vi "PYBD<-> Keyboard.vi"() -> ()   [LabVIEW 2019]
uses:
  <userlib>/MicroPython/VIs/uPythonX/uPythonX.xctl
panel:
  in  "KeyLUT":T1(xcontrol)={"Port"="PyBoard - ASRL44::INSTR", "All Code"="PLAIN = 0x00\nSHIFT = 0x02\nkbmap = dict()\nkbmap['LCTRL'] = (0x01,PLAIN)\nkbmap['LSHIFT'] = (0x02,PLAIN)\nkbmap['LALT'] = (0x04,PLAIN)\nkbmap['LMETA'] = (0x08,PLAIN)\nkbmap['RCTRL'] = (0x10,PLAIN)\nkbmap['RSHIFT'] = (0x20,PLAIN)\nkbmap['RALT'] = (0x40,PLAIN)\nkbmap['RMETA'] = (0x80,PLAIN)\nkbmap['NONE'] = (0x00,PLAIN)\nkbmap['ERR_OVF'] = (0x01,PLAIN)\nkbmap['a'] = (0x04,PLAIN)\nkbmap['A'] = (0x04,SHIFT)\nkbmap['b'] = (0x05,PLAIN)\nkbmap['B'] = (0x05,SHIFT)\nkbmap['c'] = (0x06,PLAIN)\nkbmap['C'] = (0x06,SHIFT)\nkbmap['d'] = (0x07,PLAIN)\nkbmap['D'] = (0x07,SHIFT)\nkbmap['e'] = (0x08,PLAIN)\nkbmap['E'] = (0x08,SHIFT)\nkbmap['f'] = (0x09,PLAIN)\nkbmap['F'] = (0x09,SHIFT)\nkbmap['g'] = (0x0a,PLAIN)\nkbmap['G'] = (0x0a,SHIFT)\nkbmap['h'] = (0x0b,PLAIN)\nkbmap['H'] = (0x0b,SHIFT)\nkbmap['i'] = (0x0c,PLAIN)\nkbmap['I'] = (0x0c,SHIFT)\nkbmap['j'] = (0x0d,PLAIN)\nkbmap['J'] = (0x0d,SHIFT)\nkbmap['k'] = (0x0e,PLAIN)\nkbmap['K'] = (0x0e,SHIFT)\nkbmap['l'] = (0x0f,PLAIN)\nkbmap['L'] = (0x0f,SHIFT)\nkbmap['m'] = (0x10,PLAIN)\nkbmap['M'] = (0x10,SHIFT)\nkbmap['n'] = (0x11,PLAIN)\nkbmap['N'] = (0x11,SHIFT)\nkbmap['o'] = (0x12,PLAIN)\nkbmap['O'] = (0x12,SHIFT)\nkbmap['p'] = (0x13,PLAIN)\nkbmap['P'] = (0x13,SHIFT)\nkbmap['q'] = (0x14,PLAIN)\nkbmap['Q'] = (0x14,SHIFT)\nkbmap['r'] = (0x15,PLAIN)\nkbmap['R'] = (0x15,SHIFT)\nkbmap['s'] = (0x16,PLAIN)\nkbmap['S'] = (0x16,SHIFT)\nkbmap['t'] = (0x17,PLAIN)\nkbmap['T'] = (0x17,SHIFT)\nkbmap['u'] = (0x18,PLAIN)\nkbmap['U'] = (0x18,SHIFT)\nkbmap['v'] = (0x19,PLAIN)\nkbmap['V'] = (0x19,SHIFT)\nkbmap['w'] = (0x1a,PLAIN)\nkbmap['W'] = (0x1a,SHIFT)\nkbmap['x'] = (0x1b,PLAIN)\nkbmap['X'] = (0x1b,SHIFT)\nkbmap['y'] = (0x1c,PLAIN)\nkbmap['Y'] = (0x1c,SHIFT)\nkbmap['z'] = (0x1d,PLAIN)\nkbmap['Z'] = (0x1d,SHIFT)\nkbmap['1'] = (0x1e,PLAIN)\nkbmap['!'] = (0x1e,SHIFT)\nkbmap['2'] = (0x1f,PLAIN)\nkbmap['@'] = (0x1f,SHIFT)\nkbmap['3'] = (0x20,PLAIN)\nkbmap['#'] = (0x20,SHIFT)\nkbmap['4'] = (0x21,PLAIN)\nkbmap['$'] = (0x21,SHIFT)\nkbmap['5'] = (0x22,PLAIN)\nkbmap['%'] = (0x22,SHIFT)\nkbmap['6'] = (0x23,PLAIN)\nkbmap['^'] = (0x23,SHIFT)\nkbmap['7'] = (0x24,PLAIN)\nkbmap['&'] = (0x24,SHIFT)\nkbmap['8'] = (0x25,PLAIN)\nkbmap['*'] = (0x25,SHIFT)\nkbmap['9'] = (0x26,PLAIN)\nkbmap['('] = (0x26,SHIFT)\nkbmap['0'] = (0x27,PLAIN)\nkbmap[')'] = (0x27,SHIFT)\nkbmap['ENTER'] = (0x28,PLAIN)\nkbmap['ESC'] = (0x29,PLAIN)\nkbmap['BACKSPACE'] = (0x2a,PLAIN)\nkbmap['\\t'] = (0x2b,PLAIN)\nkbmap[' '] = (0x2c,PLAIN)\nkbmap['-'] = (0x2d,PLAIN)\nkbmap['_'] = (0x2d,SHIFT)\nkbmap['='] = (0x2e,PLAIN)\nkbmap['+'] = (0x2e,SHIFT)\nkbmap['['] = (0x2f,PLAIN)\nkbmap['{'] = (0x2f,SHIFT)\nkbmap[']'] = (0x30,PLAIN)\nkbmap['}'] = (0x30,SHIFT)\nkbmap['\\\\'] = (0x31,PLAIN)\nkbmap['|'] = (0x31,SHIFT)\nkbmap['~'] = (0x32,PLAIN)\nkbmap[';'] = (0x33,PLAIN)\nkbmap[':'] = (0x33,SHIFT)\nkbmap[\"'\"] = (0x34,PLAIN)\nkbmap['\"'] = (0x34,SHIFT)\nkbmap['GRAVE'] = (0x35,PLAIN)\nkbmap[','] = (0x36,PLAIN)\nkbmap['<'] = (0x36,SHIFT)\nkbmap['.'] = (0x37,PLAIN)\nkbmap['>'] = (0x37,SHIFT)\nkbmap['/'] = (0x38,PLAIN)\nkbmap['?'] = (0x38,SHIFT)\nkbmap['CAPSLOCK'] = (0x39,PLAIN)\nkbmap['F1'] = (0x3a,PLAIN)\nkbmap['F2'] = (0x3b,PLAIN)\nkbmap['F3'] = (0x3c,PLAIN)\nkbmap['F4'] = (0x3d,PLAIN)\nkbmap['F5'] = (0x3e,PLAIN)\nkbmap['F6'] = (0x3f,PLAIN)\nkbmap['F7'] = (0x40,PLAIN)\nkbmap['F8'] = (0x41,PLAIN)\nkbmap['F9'] = (0x42,PLAIN)\nkbmap['F10'] = (0x43,PLAIN)\nkbmap['F11'] = (0x44,PLAIN)\nkbmap['F12'] = (0x45,PLAIN)\nkbmap['SYSRQ'] = (0x46,PLAIN)\nkbmap['SCROLLLOCK'] = (0x47,PLAIN)\nkbmap['PAUSE'] = (0x48,PLAIN)\nkbmap['INSERT'] = (0x49,PLAIN)\nkbmap['HOME'] = (0x4a,PLAIN)\nkbmap['PAGEUP'] = (0x4b,PLAIN)\nkbmap['DELETE'] = (0x4c,PLAIN)\nkbmap['END'] = (0x4d,PLAIN)\nkbmap['PAGEDOWN'] = (0x4e,PLAIN)\nkbmap['RIGHT'] = (0x4f,PLAIN)\nkbmap['LEFT'] = (0x50,PLAIN)\nkbmap['DOWN'] = (0x51,PLAIN)\nkbmap['UP'] = (0x52,PLAIN)\nkbmap['NUMLOCK'] = (0x53,PLAIN)\nkbmap['F13'] = (0x68,PLAIN)\nkbmap['F14'] = (0x69,PLAIN)\nkbmap['F15'] = (0x6a,PLAIN)\nkbmap['F16'] = (0x6b,PLAIN)\nkbmap['F17'] = (0x6c,PLAIN)\nkbmap['F18'] = (0x6d,PLAIN)\nkbmap['F19'] = (0x6e,PLAIN)\nkbmap['F20'] = (0x6f,PLAIN)\nkbmap['F21'] = (0x70,PLAIN)\nkbmap['F22'] = (0x71,PLAIN)\nkbmap['F23'] = (0x72,PLAIN)\nkbmap['F24'] = (0x73,PLAIN)\nkbmap['OPEN'] = (0x74,PLAIN)\nkbmap['HELP'] = (0x75,PLAIN)\nkbmap['PROPS'] = (0x76,PLAIN)\nkbmap['FRONT'] = (0x77,PLAIN)\nkbmap['STOP'] = (0x78,PLAIN)\nkbmap['AGAIN'] = (0x79,PLAIN)\nkbmap['UNDO'] = (0x7a,PLAIN)\nkbmap['CUT'] = (0x7b,PLAIN)\nkbmap['COPY'] = (0x7c,PLAIN)\nkbmap['PASTE'] = (0x7d,PLAIN)\nkbmap['FIND'] = (0x7e,PLAIN)\nkbmap['MUTE'] = (0x7f,PLAIN)\nkbmap['VOLUMEUP'] = (0x80,PLAIN)\nkbmap['VOLUMEDOWN'] = (0x81,PLAIN)"}
  out "regular expression":string="PLAIN = 0x00\nSHIFT = 0x02\nkbmap = dict()\nkbmap['MOD_LCTRL'] = (0x01,PLAIN)\nkbmap['MOD_LSHIFT'] = (0x02,PLAIN)\nkbmap['MOD_LALT'] = (0x04,PLAIN)\nkbmap['MOD_LMETA'] = (0x08,PLAIN)\nkbmap['MOD_RCTRL'] = (0x10,PLAIN)\nkbmap['MOD_RSHIFT'] = (0x20,PLAIN)\nkbmap['MOD_RALT'] = (0x40,PLAIN)\nkbmap['MOD_RMETA'] = (0x80,PLAIN)\nkbmap['NONE'] = (0x00,PLAIN)\nkbmap['ERR_OVF'] = (0x01,PLAIN)\nkbmap['a'] = (0x04,PLAIN)\nkbmap['A'] = (0x04,SHIFT)\nkbmap['b'] = (0x05,PLAIN)\nkbmap['B'] = (0x05,SHIFT)\nkbmap['c'] = (0x06,PLAIN)\nkbmap['C'] = (0x06,SHIFT)\nkbmap['d'] = (0x07,PLAIN)\nkbmap['D'] = (0x07,SHIFT)\nkbmap['e'] = (0x08,PLAIN)\nkbmap['E'] = (0x08,SHIFT)\nkbmap['f'] = (0x09,PLAIN)\nkbmap['F'] = (0x09,SHIFT)\nkbmap['g'] = (0x0a,PLAIN)\nkbmap['G'] = (0x0a,SHIFT)\nkbmap['h'] = (0x0b,PLAIN)\nkbmap['H'] = (0x0b,SHIFT)\nkbmap['i'] = (0x0c,PLAIN)\nkbmap['I'] = (0x0c,SHIFT)\nkbmap['j'] = (0x0d,PLAIN)\nkbmap['J'] = (0x0d,SHIFT)\nkbmap['k'] = (0x0e,PLAIN)\nkbmap['K'] = (0x0e,SHIFT)\nkbmap['l'] = (0x0f,PLAIN)\nkbmap['L'] = (0x0f,SHIFT)\nkbmap['m'] = (0x10,PLAIN)\nkbmap['M'] = (0x10,SHIFT)\nkbmap['n'] = (0x11,PLAIN)\nkbmap['N'] = (0x11,SHIFT)\nkbmap['o'] = (0x12,PLAIN)\nkbmap['O'] = (0x12,SHIFT)\nkbmap['p'] = (0x13,PLAIN)\nkbmap['P'] = (0x13,SHIFT)\nkbmap['q'] = (0x14,PLAIN)\nkbmap['Q'] = (0x14,SHIFT)\nkbmap['r'] = (0x15,PLAIN)\nkbmap['R'] = (0x15,SHIFT)\nkbmap['s'] = (0x16,PLAIN)\nkbmap['S'] = (0x16,SHIFT)\nkbmap['t'] = (0x17,PLAIN)\nkbmap['T'] = (0x17,SHIFT)\nkbmap['u'] = (0x18,PLAIN)\nkbmap['U'] = (0x18,SHIFT)\nkbmap['v'] = (0x19,PLAIN)\nkbmap['V'] = (0x19,SHIFT)\nkbmap['w'] = (0x1a,PLAIN)\nkbmap['W'] = (0x1a,SHIFT)\nkbmap['x'] = (0x1b,PLAIN)\nkbmap['X'] = (0x1b,SHIFT)\nkbmap['y'] = (0x1c,PLAIN)\nkbmap['Y'] = (0x1c,SHIFT)\nkbmap['z'] = (0x1d,PLAIN)\nkbmap['Z'] = (0x1d,SHIFT)\nkbmap['1'] = (0x1e,PLAIN)\nkbmap['1'] = (0x1e,SHIFT)\nkbmap['2'] = (0x1f,PLAIN)\nkbmap['2'] = (0x1f,SHIFT)\nkbmap['3'] = (0x20,PLAIN)\nkbmap['3'] = (0x20,SHIFT)\nkbmap['4'] = (0x21,PLAIN)\nkbmap['4'] = (0x21,SHIFT)\nkbmap['5'] = (0x22,PLAIN)\nkbmap['5'] = (0x22,SHIFT)\nkbmap['6'] = (0x23,PLAIN)\nkbmap['6'] = (0x23,SHIFT)\nkbmap['7'] = (0x24,PLAIN)\nkbmap['7'] = (0x24,SHIFT)\nkbmap['8'] = (0x25,PLAIN)\nkbmap['8'] = (0x25,SHIFT)\nkbmap['9'] = (0x26,PLAIN)\nkbmap['9'] = (0x26,SHIFT)\nkbmap['0'] = (0x27,PLAIN)\nkbmap['0'] = (0x27,SHIFT)\nkbmap['ENTER'] = (0x28,PLAIN)\nkbmap['ESC'] = (0x29,PLAIN)\nkbmap['BACKSPACE'] = (0x2a,PLAIN)\nkbmap['TAB'] = (0x2b,PLAIN)\nkbmap['SPACE'] = (0x2c,PLAIN)\nkbmap['MINUS'] = (0x2d,PLAIN)\nkbmap['EQUAL'] = (0x2e,PLAIN)\nkbmap['LEFTBRACE'] = (0x2f,PLAIN)\nkbmap['RIGHTBRACE'] = (0x30,PLAIN)\nkbmap['BACKSLASH'] = (0x31,PLAIN)\nkbmap['HASHTILDE'] = (0x32,PLAIN)\nkbmap['SEMICOLON'] = (0x33,PLAIN)\nkbmap['APOSTROPHE'] = (0x34,PLAIN)\nkbmap['GRAVE'] = (0x35,PLAIN)\nkbmap['COMMA'] = (0x36,PLAIN)\nkbmap['DOT'] = (0x37,PLAIN)\nkbmap['SLASH'] = (0x38,PLAIN)\nkbmap['CAPSLOCK'] = (0x39,PLAIN)\nkbmap['F'] = (0x3a,PLAIN)\nkbmap['1'] = (0x3a,SHIFT)\nkbmap['F'] = (0x3b,PLAIN)\nkbmap['2'] = (0x3b,SHIFT)\nkbmap['F'] = (0x3c,PLAIN)\nkbmap['3'] = (0x3c,SHIFT)\nkbmap['F'] = (0x3d,PLAIN)\nkbmap['4'] = (0x3d,SHIFT)\nkbmap['F'] = (0x3e,PLAIN)\nkbmap['5'] = (0x3e,SHIFT)\nkbmap['F'] = (0x3f,PLAIN)\nkbmap['6'] = (0x3f,SHIFT)\nkbmap['F'] = (0x40,PLAIN)\nkbmap['7'] = (0x40,SHIFT)\nkbmap['F'] = (0x41,PLAIN)\nkbmap['8'] = (0x41,SHIFT)\nkbmap['F'] = (0x42,PLAIN)\nkbmap['9'] = (0x42,SHIFT)\nkbmap['F10'] = (0x43,PLAIN)\nkbmap['F11'] = (0x44,PLAIN)\nkbmap['F12'] = (0x45,PLAIN)\nkbmap['SYSRQ'] = (0x46,PLAIN)\nkbmap['SCROLLLOCK'] = (0x47,PLAIN)\nkbmap['PAUSE'] = (0x48,PLAIN)\nkbmap['INSERT'] = (0x49,PLAIN)\nkbmap['HOME'] = (0x4a,PLAIN)\nkbmap['PAGEUP'] = (0x4b,PLAIN)\nkbmap['DELETE'] = (0x4c,PLAIN)\nkbmap['END'] = (0x4d,PLAIN)\nkbmap['PAGEDOWN'] = (0x4e,PLAIN)\nkbmap['RIGHT'] = (0x4f,PLAIN)\nkbmap['LEFT'] = (0x50,PLAIN)\nkbmap['DOWN'] = (0x51,PLAIN)\nkbmap['U'] = (0x52,PLAIN)\nkbmap['P'] = (0x52,SHIFT)\nkbmap['NUMLOCK'] = (0x53,PLAIN)\nkbmap['KPSLASH'] = (0x54,PLAIN)\nkbmap['KPASTERISK'] = (0x55,PLAIN)\nkbmap['KPMINUS'] = (0x56,PLAIN)\nkbmap['KPPLUS'] = (0x57,PLAIN)\nkbmap['KPENTER'] = (0x58,PLAIN)\nkbmap['KP1'] = (0x59,PLAIN)\nkbmap['KP2'] = (0x5a,PLAIN)\nkbmap['KP3'] = (0x5b,PLAIN)\nkbmap['KP4'] = (0x5c,PLAIN)\nkbmap['KP5'] = (0x5d,PLAIN)\nkbmap['KP6'] = (0x5e,PLAIN)\nkbmap['KP7'] = (0x5f,PLAIN)\nkbmap['KP8'] = (0x60,PLAIN)\nkbmap['KP9'] = (0x61,PLAIN)\nkbmap['KP0'] = (0x62,PLAIN)\nkbmap['KPDOT'] = (0x63,PLAIN)\nkbmap['102ND'] = (0x64,PLAIN)\nkbmap['COMPOSE'] = (0x65,PLAIN)\nkbmap['POWER'] = (0x66,PLAIN)\nkbmap['KPEQUAL'] = (0x67,PLAIN)\nkbmap['F13'] = (0x68,PLAIN)\nkbmap['F14'] = (0x69,PLAIN)\nkbmap['F15'] = (0x6a,PLAIN)\nkbmap['F16'] = (0x6b,PLAIN)\nkbmap['F17'] = (0x6c,PLAIN)\nkbmap['F18'] = (0x6d,PLAIN)\nkbmap['F19'] = (0x6e,PLAIN)\nkbmap['F20'] = (0x6f,PLAIN)\nkbmap['F21'] = (0x70,PLAIN)\nkbmap['F22'] = (0x71,PLAIN)\nkbmap['F23'] = (0x72,PLAIN)\nkbmap['F24'] = (0x73,PLAIN)\nkbmap['OPEN'] = (0x74,PLAIN)\nkbmap['HELP'] = (0x75,PLAIN)\nkbmap['PROPS'] = (0x76,PLAIN)\nkbmap['FRONT'] = (0x77,PLAIN)\nkbmap['STOP'] = (0x78,PLAIN)\nkbmap['AGAIN'] = (0x79,PLAIN)\nkbmap['UNDO'] = (0x7a,PLAIN)\nkbmap['CUT'] = (0x7b,PLAIN)\nkbmap['COPY'] = (0x7c,PLAIN)\nkbmap['PASTE'] = (0x7d,PLAIN)\nkbmap['FIND'] = (0x7e,PLAIN)\nkbmap['MUTE'] = (0x7f,PLAIN)\nkbmap['VOLUMEUP'] = (0x80,PLAIN)\nkbmap['VOLUMEDOWN'] = (0x81,PLAIN)\n"
  out "Table Control":string[][](table)=[["MOD_LCTRL", "0x01", ""], ["MOD_LSHIFT", "0x02", ""], ["MOD_LALT", "0x04", ""], ["MOD_LMETA", "0x08", ""], ["MOD_RCTRL", "0x10", ""], ["MOD_RSHIFT", "0x20", ""], ["MOD_RALT", "0x40", ""], ["MOD_RMETA", "0x80", ""], ["NONE", "0x00", "No key pressed"], ["ERR_OVF", "0x01", "Keyboard Error Roll Over - used for all slots if too many keys are pressed (\"Phantom key\")"], ["A", "0x04", "Keyboard a and A"], ["B", "0x05", "Keyboard b and B"], ["C", "0x06", "Keyboard c and C"], ["D", "0x07", "Keyboard d and D"], ["E", "0x08", "Keyboard e and E"], ["F", "0x09", "Keyboard f and F"], ["G", "0x0a", "Keyboard g and G"], ["H", "0x0b", "Keyboard h and H"], ["I", "0x0c", "Keyboard i and I"], ["J", "0x0d", "Keyboard j and J"], ["K", "0x0e", "Keyboard k and K"], ["L", "0x0f", "Keyboard l and L"], ["M", "0x10", "Keyboard m and M"], ["N", "0x11", "Keyboard n and N"], ["O", "0x12", "Keyboard o and O"], ["P", "0x13", "Keyboard p and P"], ["Q", "0x14", "Keyboard q and Q"], ["R", "0x15", "Keyboard r and R"], ["S", "0x16", "Keyboard s and S"], ["T", "0x17", "Keyboard t and T"], ["U", "0x18", "Keyboard u and U"], ["V", "0x19", "Keyboard v and V"], ["W", "0x1a", "Keyboard w and W"], ["X", "0x1b", "Keyboard x and X"], ["Y", "0x1c", "Keyboard y and Y"], ["Z", "0x1d", "Keyboard z and Z"], ["1", "0x1e", "Keyboard 1 and !"], ["2", "0x1f", "Keyboard 2 and @"], ["3", "0x20", "Keyboard 3 and #"], ["4", "0x21", "Keyboard 4 and $"], ["5", "0x22", "Keyboard 5 and %"], ["6", "0x23", "Keyboard 6 and ^"], ["7", "0x24", "Keyboard 7 and &"], ["8", "0x25", "Keyboard 8 and *"], ["9", "0x26", "Keyboard 9 and ("], ["0", "0x27", "Keyboard 0 and )"], ["ENTER", "0x28", "Keyboard Return (ENTER)"], ["ESC", "0x29", "Keyboard ESCAPE"], ["BACKSPACE", "0x2a", "Keyboard DELETE (Backspace)"], ["TAB", "0x2b", "Keyboard Tab"], ["SPACE", "0x2c", "Keyboard Spacebar"], ["MINUS", "0x2d", "Keyboard - and _"], ["EQUAL", "0x2e", "Keyboard = and +"], ["LEFTBRACE", "0x2f", "Keyboard [ and {"], ["RIGHTBRACE", "0x30", "Keyboard ] and }"], ["BACKSLASH", "0x31", "Keyboard \\ and |"], ["HASHTILDE", "0x32", "Keyboard Non-US # and ~"], ["SEMICOLON", "0x33", "Keyboard ; and :"], ["APOSTROPHE", "0x34", "Keyboard ' and \""], ["GRAVE", "0x35", "Keyboard ` and ~"], ["COMMA", "0x36", "Keyboard , and <"], ["DOT", "0x37", "Keyboard . and >"], ["SLASH", "0x38", "Keyboard / and ?"], ["CAPSLOCK", "0x39", "Keyboard Caps Lock"], ["F1", "0x3a", "Keyboard F1"], ["F2", "0x3b", "Keyboard F2"], ["F3", "0x3c", "Keyboard F3"], ["F4", "0x3d", "Keyboard F4"], ["F5", "0x3e", "Keyboard F5"], ["F6", "0x3f", "Keyboard F6"], ["F7", "0x40", "Keyboard F7"], ["F8", "0x41", "Keyboard F8"], ["F9", "0x42", "Keyboard F9"], ["F10", "0x43", "Keyboard F10"], ["F11", "0x44", "Keyboard F11"], ["F12", "0x45", "Keyboard F12"], ["SYSRQ", "0x46", "Keyboard Print Screen"], ["SCROLLLOCK", "0x47", "Keyboard Scroll Lock"], ["PAUSE", "0x48", "Keyboard Pause"], ["INSERT", "0x49", "Keyboard Insert"], ["HOME", "0x4a", "Keyboard Home"], ["PAGEUP", "0x4b", "Keyboard Page Up"], ["DELETE", "0x4c", "Keyboard Delete Forward"], ["END", "0x4d", "Keyboard End"], ["PAGEDOWN", "0x4e", "Keyboard Page Down"], ["RIGHT", "0x4f", "Keyboard Right Arrow"], ["LEFT", "0x50", "Keyboard Left Arrow"], ["DOWN", "0x51", "Keyboard Down Arrow"], ["UP", "0x52", "Keyboard Up Arrow"], ["NUMLOCK", "0x53", "Keyboard Num Lock and Clear"], ["KPSLASH", "0x54", "Keypad /"], ["KPASTERISK", "0x55", "Keypad *"], ["KPMINUS", "0x56", "Keypad -"], ["KPPLUS", "0x57", "Keypad +"], ["KPENTER", "0x58", "Keypad ENTER"], ["KP1", "0x59", "Keypad 1 and End"], ["KP2", "0x5a", "Keypad 2 and Down Arrow"], ["KP3", "0x5b", "Keypad 3 and PageDn"], ["KP4", "0x5c", "Keypad 4 and Left Arrow"], ["KP5", "0x5d", "Keypad 5"], ["KP6", "0x5e", "Keypad 6 and Right Arrow"], ["KP7", "0x5f", "Keypad 7 and Home"], ["KP8", "0x60", "Keypad 8 and Up Arrow"], ["KP9", "0x61", "Keypad 9 and Page Up"], ["KP0", "0x62", "Keypad 0 and Insert"], ["KPDOT", "0x63", "Keypad . and Delete"], ["102ND", "0x64", "Keyboard Non-US \\ and |"], ["COMPOSE", "0x65", "Keyboard Application"], ["POWER", "0x66", "Keyboard Power"], ["KPEQUAL", "0x67", "Keypad ="], ["F13", "0x68", "Keyboard F13"], ["F14", "0x69", "Keyboard F14"], ["F15", "0x6a", "Keyboard F15"], ["F16", "0x6b", "Keyboard F16"], ["F17", "0x6c", "Keyboard F17"], ["F18", "0x6d", "Keyboard F18"], ["F19", "0x6e", "Keyboard F19"], ["F20", "0x6f", "Keyboard F20"], ["F21", "0x70", "Keyboard F21"], ["F22", "0x71", "Keyboard F22"], ["F23", "0x72", "Keyboard F23"], ["F24", "0x73", "Keyboard F24"], ["OPEN", "0x74", "Keyboard Execute"], ["HELP", "0x75", "Keyboard Help"], ["PROPS", "0x76", "Keyboard Menu"], ["FRONT", "0x77", "Keyboard Select"], ["STOP", "0x78", "Keyboard Stop"], ["AGAIN", "0x79", "Keyboard Again"], ["UNDO", "0x7a", "Keyboard Undo"], ["CUT", "0x7b", "Keyboard Cut"], ["COPY", "0x7c", "Keyboard Copy"], ["PASTE", "0x7d", "Keyboard Paste"], ["FIND", "0x7e", "Keyboard Find"], ["MUTE", "0x7f", "Keyboard Mute"], ["VOLUMEUP", "0x80", "Keyboard Volume Up"], ["VOLUMEDOWN", "0x81", "Keyboard Volume Downe"]]
  in  "uPythonX":T1(xcontrol)={"Port"="PyBoard - ASRL44::INSTR", "All Code"="'''\nhttp://wiki.micropython.org/USB-HID-Keyboard-mode-example-a-password-dongle\n     \n#boot.py\nimport machine\nimport pyb\n#pyb.main('main.py') # main script to run after this one\n#pyb.usb_mode('CDC+MSC') # act as a serial and a storage device\npyb.usb_mode('CDC+HID',hid=pyb.hid_keyboard)\n\nFor arduino - https://www.sparkfun.com/tutorials/337\n'''\n\nimport pyb,utime\nimport KeyLUT\nkb = pyb.USB_HID()\nbuf = bytearray(8)\n# Sending T\n# Do the key down\ndef typeKey(letter):\n     \n     buf[0] = KeyLUT.kbmap[letter][1]\n     buf[2] = KeyLUT.kbmap[letter][0]\n     kb.send(buf)\n     pyb.delay(20)\n     # Do the key up\n     buf[0] = 0x00\n     buf[2] = 0x00\n     kb.send(buf)\n     pyb.delay(20)     \n\ndef typeKeys(string):\n     for letter in string:\n          typeKey(letter)\n          \ntypeKeys('!@#$%^&*(): I have a _+=-34?/<>,')"}
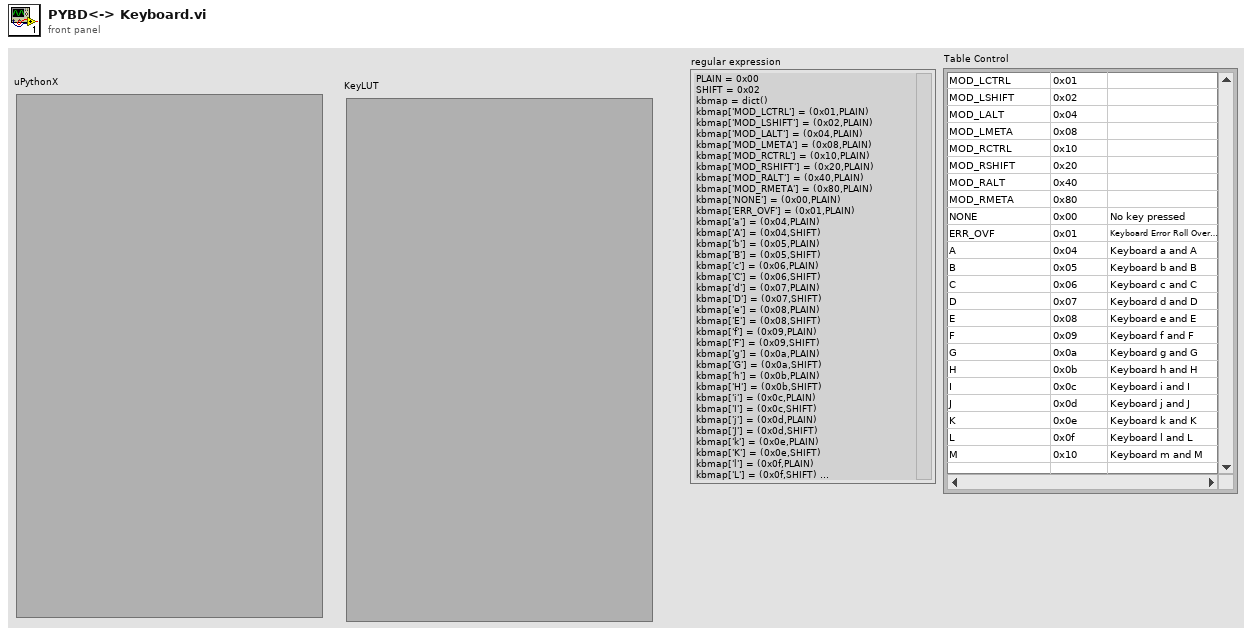
[diagram p1: front panel]
types:
  T1 = cluster{"Port":refnum<visa-resource-name>, "All Code":string}
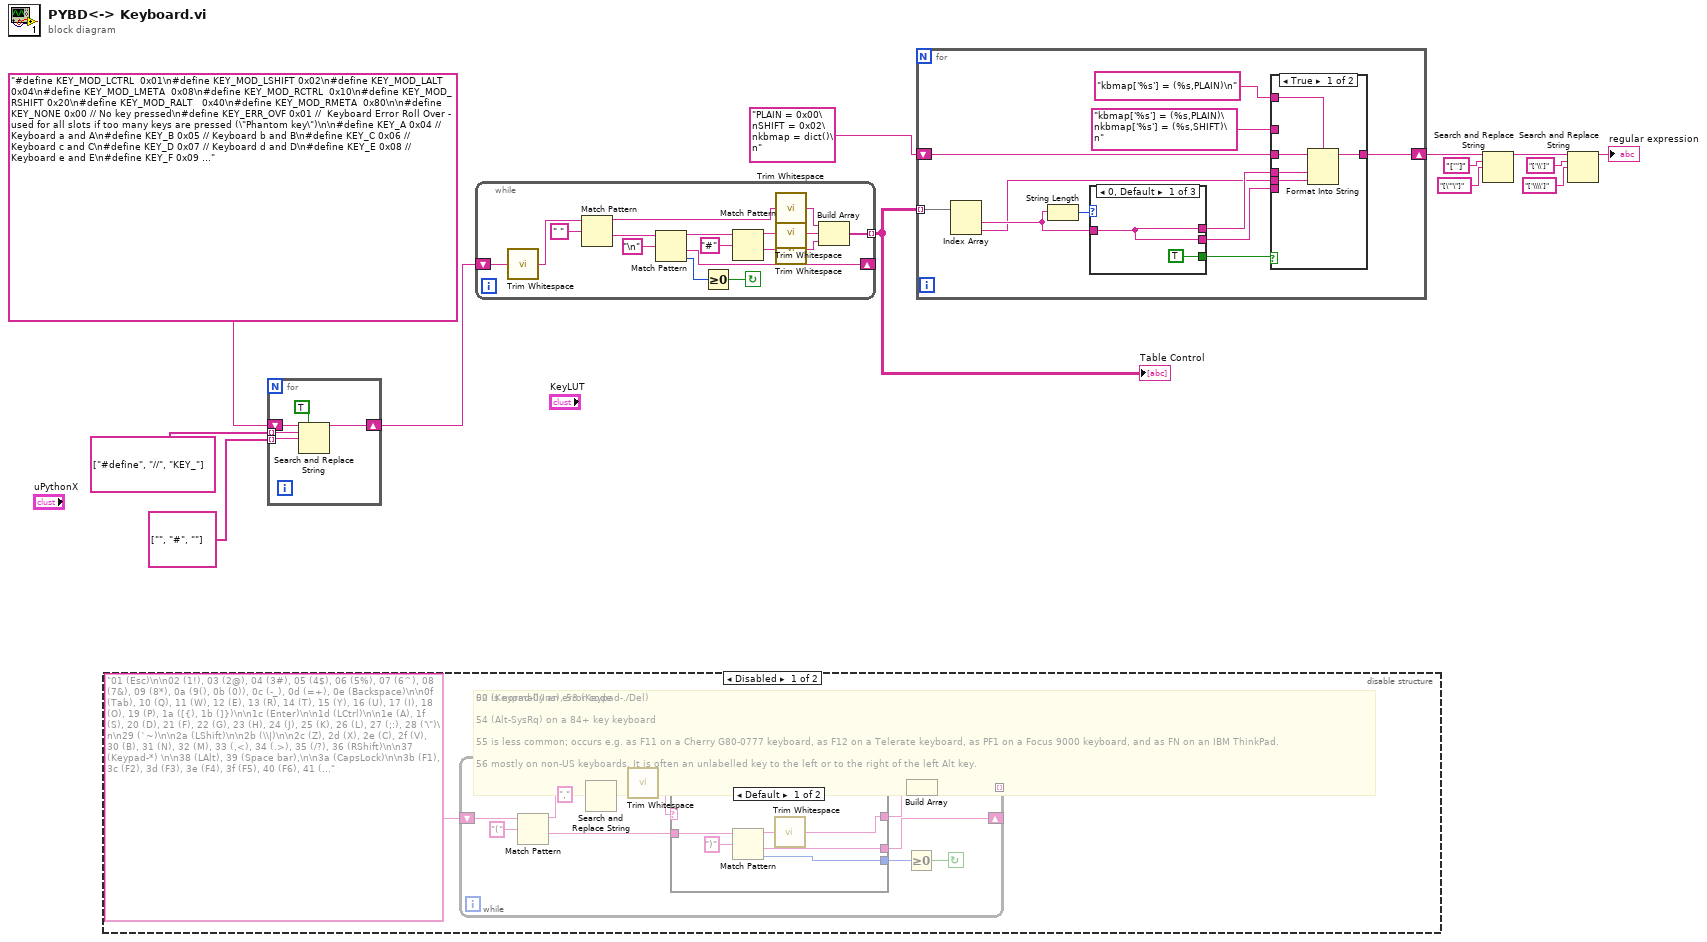
[diagram p0: block diagram]
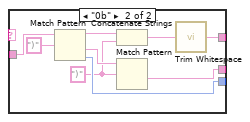
[diagram p2: hidden frame]
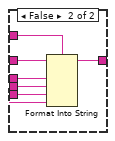
[diagram p4: hidden frame]
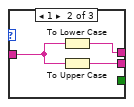
[diagram p5: hidden frame]
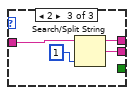
[diagram p6: hidden frame]
diagram:
  n1 = disable-structure shown="Disabled" {
    frame Disabled {
      # "00 is normally an error code"
      # "52 (Keypad-0/Ins), 53 (Keypad-./Del)\n\n54 (Alt-SysRq) on a 84+ key keyboard\n\n55 is less common; occurs e.g. as F11 on a Cherry G80-0777 keyboard, as F12 on a Telerate keyboard, as PF1 on a Focus 9000 keyboard, and as FN on an IBM ThinkPad.\n\n56 mostly on non-US keyboards. It is often an unlabelled key to the left or to the right of the left Alt key."
      n2 = while {
        shift-right: [w23] -> _
        shift-left: "01 (Esc)\n\n02 (1!), 03 (2@), 04 (3#), 05 (4$), 06 (5%), 07 (6^), 08 (7&), 09 (8*), 0a (9(), 0b (0)), 0c (-_), 0d (=+), 0e (Backspace)\n\n0f (Tab), 10 (Q), 11 (W), 12 (E), 13 (R), 14 (T), 15 (Y), 16 (U), 17 (I), 18 (O), 19 (P), 1a ([{), 1b (]})\n\n1c (Enter)\n\n1d (LCtrl)\n\n1e (A), 1f (S), 20 (D), 21 (F), 22 (G), 23 (H), 24 (J), 25 (K), 26 (L), 27 (;:), 28 ('\")\n\n29 (`~)\n\n2a (LShift)\n\n2b (\\|)\n\n2c (Z), 2d (X), 2e (C), 2f (V), 30 (B), 31 (N), 32 (M), 33 (,<), 34 (.>), 35 (/?), 36 (RShift)\n\n37 (Keypad-*) \n\n38 (LAlt), 39 (Space bar),\n\n3a (CapsLock)\n\n3b (F1), 3c (F2), 3d (F3), 3e (F4), 3f (F5), 40 (F6), 41 (F7), 42 (F8), 43 (F9), 44 (F10)\n\n45 (NumLock)\n\n46 (ScrollLock)\n\n47 (Keypad-7/Home), 48 (Keypad-8/Up), 49 (Keypad-9/PgUp)\n\n4a (Keypad--)\n\n4b (Keypad-4/Left), 4c (Keypad-5), 4d (Keypad-6/Right), 4e (Keypad-+)\n\n4f (Keypad-1/End), 50 (Keypad-2/Down), 51 (Keypad-3/PgDn)\n" ("String") -> [w26]
        tunnel: [w19] -> _ mode=indexing
        stop <- w21 continue-if-true
        n3 = Match Pattern(string=w26, regular expression="(") -> (before substring=w18:string, after substring=w24:string)  [unwired: 1 in, 2 out]
        n4 = Search and Replace String(input string=w18, search string="," ("regular expression")) -> (result string=w16:string)  [unwired: 6 in, 3 out]
        n5 = call <vilib>:"Trim Whitespace.vi"("string"=w16) -> ("trimmed string"=w15:string)  [unwired: 1 in]
        n6 = case shown="Default" w15 {
          tunnel: w24 -> [w32 w41]
          tunnel: [w29 w36] -> w23
          tunnel: [w28 w39] -> w22
          tunnel: [w27 w38] -> w20
          frame Default {
            n7 = Match Pattern(string=w32, regular expression=")") -> (before substring=w30:string, after substring=w29:string, offset past match=w28:i32)  [unwired: 1 in, 1 out]
            n8 = call <vilib>:"Trim Whitespace.vi"("string"=w30) -> ("trimmed string"=w27:string)  [unwired: 1 in]
          }
          frame "0b" {
            w34 = ")" ("regular expression")
            n9 = Match Pattern(string=w41, regular expression=")") -> (before substring=w35:string, after substring=w37:string, offset past match=w39:i32)  [unwired: 1 in, 1 out]
            n10 = Concatenate Strings(w35, w34) -> (w33:string)
            n11 = Match Pattern(string=w37, regular expression=w34) -> (after substring=w36:string)  [unwired: 1 in, 3 out]
            n12 = call <vilib>:"Trim Whitespace.vi"("string"=w33) -> ("trimmed string"=w38:string)  [unwired: 1 in]
          }
        }
        n13 = Greater Or Equal To 0?(x=w22) -> (x >= 0?=w21:bool)
        n14 = Build Array(w15, w20) -> (w19:string[])
      }
    }
    frame Enabled {
    }
  }
  n15 = for {
    tunnel: string[] ["#define", "//", "KEY_"] -> [w45] mode=indexing
    tunnel: string[] ["", "#", ""] -> [w44] mode=indexing
    shift-right: [w42] -> w1
    shift-left: "#define KEY_MOD_LCTRL  0x01\n#define KEY_MOD_LSHIFT 0x02\n#define KEY_MOD_LALT   0x04\n#define KEY_MOD_LMETA  0x08\n#define KEY_MOD_RCTRL  0x10\n#define KEY_MOD_RSHIFT 0x20\n#define KEY_MOD_RALT   0x40\n#define KEY_MOD_RMETA  0x80\n\n#define KEY_NONE 0x00 // No key pressed\n#define KEY_ERR_OVF 0x01 //  Keyboard Error Roll Over - used for all slots if too many keys are pressed (\"Phantom key\")\n\n#define KEY_A 0x04 // Keyboard a and A\n#define KEY_B 0x05 // Keyboard b and B\n#define KEY_C 0x06 // Keyboard c and C\n#define KEY_D 0x07 // Keyboard d and D\n#define KEY_E 0x08 // Keyboard e and E\n#define KEY_F 0x09 // Keyboard f and F\n#define KEY_G 0x0a // Keyboard g and G\n#define KEY_H 0x0b // Keyboard h and H\n#define KEY_I 0x0c // Keyboard i and I\n#define KEY_J 0x0d // Keyboard j and J\n#define KEY_K 0x0e // Keyboard k and K\n#define KEY_L 0x0f // Keyboard l and L\n#define KEY_M 0x10 // Keyboard m and M\n#define KEY_N 0x11 // Keyboard n and N\n#define KEY_O 0x12 // Keyboard o and O\n#define KEY_P 0x13 // Keyboard p and P\n#define KEY_Q 0x14 // Keyboard q and Q\n#define KEY_R 0x15 // Keyboard r and R\n#define KEY_S 0x16 // Keyboard s and S\n#define KEY_T 0x17 // Keyboard t and T\n#define KEY_U 0x18 // Keyboard u and U\n#define KEY_V 0x19 // Keyboard v and V\n#define KEY_W 0x1a // Keyboard w and W\n#define KEY_X 0x1b // Keyboard x and X\n#define KEY_Y 0x1c // Keyboard y and Y\n#define KEY_Z 0x1d // Keyboard z and Z\n\n#define KEY_1 0x1e // Keyboard 1 and !\n#define KEY_2 0x1f // Keyboard 2 and @\n#define KEY_3 0x20 // Keyboard 3 and #\n#define KEY_4 0x21 // Keyboard 4 and $\n#define KEY_5 0x22 // Keyboard 5 and %\n#define KEY_6 0x23 // Keyboard 6 and ^\n#define KEY_7 0x24 // Keyboard 7 and &\n#define KEY_8 0x25 // Keyboard 8 and *\n#define KEY_9 0x26 // Keyboard 9 and (\n#define KEY_0 0x27 // Keyboard 0 and )\n\n#define KEY_ENTER 0x28 // Keyboard Return (ENTER)\n#define KEY_ESC 0x29 // Keyboard ESCAPE\n#define KEY_BACKSPACE 0x2a // Keyboard DELETE (Backspace)\n#define KEY_TAB 0x2b // Keyboard Tab\n#define KEY_SPACE 0x2c // Keyboard Spacebar\n#define KEY_MINUS 0x2d // Keyboard - and _\n#define KEY_EQUAL 0x2e // Keyboard = and +\n#define KEY_LEFTBRACE 0x2f // Keyboard [ and {\n#define KEY_RIGHTBRACE 0x30 // Keyboard ] and }\n#define KEY_BACKSLASH 0x31 // Keyboard \\ and |\n#define KEY_HASHTILDE 0x32 // Keyboard Non-US # and ~\n#define KEY_SEMICOLON 0x33 // Keyboard ; and :\n#define KEY_APOSTROPHE 0x34 // Keyboard ' and \"\n#define KEY_GRAVE 0x35 // Keyboard ` and ~\n#define KEY_COMMA 0x36 // Keyboard , and <\n#define KEY_DOT 0x37 // Keyboard . and >\n#define KEY_SLASH 0x38 // Keyboard / and ?\n#define KEY_CAPSLOCK 0x39 // Keyboard Caps Lock\n\n#define KEY_F1 0x3a // Keyboard F1\n#define KEY_F2 0x3b // Keyboard F2\n#define KEY_F3 0x3c // Keyboard F3\n#define KEY_F4 0x3d // Keyboard F4\n#define KEY_F5 0x3e // Keyboard F5\n#define KEY_F6 0x3f // Keyboard F6\n#define KEY_F7 0x40 // Keyboard F7\n#define KEY_F8 0x41 // Keyboard F8\n#define KEY_F9 0x42 // Keyboard F9\n#define KEY_F10 0x43 // Keyboard F10\n#define KEY_F11 0x44 // Keyboard F11\n#define KEY_F12 0x45 // Keyboard F12\n\n#define KEY_SYSRQ 0x46 // Keyboard Print Screen\n#define KEY_SCROLLLOCK 0x47 // Keyboard Scroll Lock\n#define KEY_PAUSE 0x48 // Keyboard Pause\n#define KEY_INSERT 0x49 // Keyboard Insert\n#define KEY_HOME 0x4a // Keyboard Home\n#define KEY_PAGEUP 0x4b // Keyboard Page Up\n#define KEY_DELETE 0x4c // Keyboard Delete Forward\n#define KEY_END 0x4d // Keyboard End\n#define KEY_PAGEDOWN 0x4e // Keyboard Page Down\n#define KEY_RIGHT 0x4f // Keyboard Right Arrow\n#define KEY_LEFT 0x50 // Keyboard Left Arrow\n#define KEY_DOWN 0x51 // Keyboard Down Arrow\n#define KEY_UP 0x52 // Keyboard Up Arrow\n\n#define KEY_NUMLOCK 0x53 // Keyboard Num Lock and Clear\n#define KEY_KPSLASH 0x54 // Keypad /\n#define KEY_KPASTERISK 0x55 // Keypad *\n#define KEY_KPMINUS 0x56 // Keypad -\n#define KEY_KPPLUS 0x57 // Keypad +\n#define KEY_KPENTER 0x58 // Keypad ENTER\n#define KEY_KP1 0x59 // Keypad 1 and End\n#define KEY_KP2 0x5a // Keypad 2 and Down Arrow\n#define KEY_KP3 0x5b // Keypad 3 and PageDn\n#define KEY_KP4 0x5c // Keypad 4 and Left Arrow\n#define KEY_KP5 0x5d // Keypad 5\n#define KEY_KP6 0x5e // Keypad 6 and Right Arrow\n#define KEY_KP7 0x5f // Keypad 7 and Home\n#define KEY_KP8 0x60 // Keypad 8 and Up Arrow\n#define KEY_KP9 0x61 // Keypad 9 and Page Up\n#define KEY_KP0 0x62 // Keypad 0 and Insert\n#define KEY_KPDOT 0x63 // Keypad . and Delete\n\n#define KEY_102ND 0x64 // Keyboard Non-US \\ and |\n#define KEY_COMPOSE 0x65 // Keyboard Application\n#define KEY_POWER 0x66 // Keyboard Power\n#define KEY_KPEQUAL 0x67 // Keypad =\n\n#define KEY_F13 0x68 // Keyboard F13\n#define KEY_F14 0x69 // Keyboard F14\n#define KEY_F15 0x6a // Keyboard F15\n#define KEY_F16 0x6b // Keyboard F16\n#define KEY_F17 0x6c // Keyboard F17\n#define KEY_F18 0x6d // Keyboard F18\n#define KEY_F19 0x6e // Keyboard F19\n#define KEY_F20 0x6f // Keyboard F20\n#define KEY_F21 0x70 // Keyboard F21\n#define KEY_F22 0x71 // Keyboard F22\n#define KEY_F23 0x72 // Keyboard F23\n#define KEY_F24 0x73 // Keyboard F24\n\n#define KEY_OPEN 0x74 // Keyboard Execute\n#define KEY_HELP 0x75 // Keyboard Help\n#define KEY_PROPS 0x76 // Keyboard Menu\n#define KEY_FRONT 0x77 // Keyboard Select\n#define KEY_STOP 0x78 // Keyboard Stop\n#define KEY_AGAIN 0x79 // Keyboard Again\n#define KEY_UNDO 0x7a // Keyboard Undo\n#define KEY_CUT 0x7b // Keyboard Cut\n#define KEY_COPY 0x7c // Keyboard Copy\n#define KEY_PASTE 0x7d // Keyboard Paste\n#define KEY_FIND 0x7e // Keyboard Find\n#define KEY_MUTE 0x7f // Keyboard Mute\n#define KEY_VOLUMEUP 0x80 // Keyboard Volume Up\n#define KEY_VOLUMEDOWN 0x81 // Keyboard Volume Downe" ("String") -> [w46]
    n16 = Search and Replace String(replace all?=TRUE ("replace all? (F)"), input string=w46, search string=w45, replace string=w44) -> (result string=w42:string)  [unwired: 4 in, 3 out]
  }
  n17 = while {
    shift-right: [w52] -> _
    shift-left: w1 -> [w63]
    tunnel: [w58] -> w12 mode=indexing
    stop <- w60 continue-if-true
    n18 = call <vilib>:"Trim Whitespace.vi"("string"=w63) -> ("trimmed string"=w54:string)  [unwired: 1 in]
    n19 = Match Pattern(string=w54, regular expression=" ") -> (before substring=w56:string, after substring=w61:string)  [unwired: 1 in, 2 out]
    n20 = Match Pattern(string=w61, regular expression="\n") -> (before substring=w51:string, after substring=w52:string, offset past match=w47:i32)  [unwired: 1 in, 1 out]
    n21 = Greater Or Equal To 0?(x=w47) -> (x >= 0?=w60:bool)
    n22 = Match Pattern(string=w51, regular expression="#") -> (before substring=w50:string, after substring=w49:string)  [unwired: 1 in, 2 out]
    n23 = call <vilib>:"Trim Whitespace.vi"("string"=w56) -> ("trimmed string"=w57:string)  [unwired: 1 in]
    n24 = call <vilib>:"Trim Whitespace.vi"("string"=w50) -> ("trimmed string"=w59:string)  [unwired: 1 in]
    n25 = call <vilib>:"Trim Whitespace.vi"("string"=w49) -> ("trimmed string"=w48:string)  [unwired: 1 in]
    n26 = Build Array(w57, w59, w48) -> (w58:string[])
  }
  "Table Control" <- w12
  n27 = for {
    tunnel: w12 -> [w74] mode=indexing
    shift-right: [w68] -> w9
    shift-left: "PLAIN = 0x00\nSHIFT = 0x02\nkbmap = dict()\n" ("regular expression") -> [w69]
    n28 = Index Array(array=w74) -> (element #1=w65:string, element #2=w64:string)  [unwired: 2 in]
    n29 = String Length(string=w65) -> (length=w72:i32)
    n30 = case shown="0, Default" w72 {
      tunnel: w65 -> [w87 w90 w94]
      tunnel: [w87 w89 w93] -> w71
      tunnel: [w87 w88 w91] -> w70
      tunnel: [TRUE _ _] -> w67
      frame 0, Default {
      }
      frame 1 {
        n31 = To Lower Case(string=w90) -> (all lower case string=w89:string)
        n32 = To Upper Case(1:w90) -> (0:w88:string)
      }
      frame 2 {
        n33 = Search/Split String(string=w94, offset (0)=1) -> (substring before match=w93:string, match + rest of string=w91:string)  [unwired: 1 in, 1 out]
      }
    }
    n34 = case shown="True" w67 {
      tunnel: "kbmap['%s'] = (%s,PLAIN)\nkbmap['%s'] = (%s,SHIFT)\n" ("regular expression") -> [_ w85]
      tunnel: w64 -> [w79 w84]
      tunnel: w71 -> [w78 w83]
      tunnel: w70 -> [_ w82]
      tunnel: w69 -> [w77 w81]
      tunnel: [w76 w80] -> w68
      tunnel: "kbmap['%s'] = (%s,PLAIN)\n" ("regular expression") -> [w75 _]
      frame True {
        n35 = Format Into String(format string=w75, initial string=w77, w78, w79) -> (resulting string=w76:string)  [unwired: 1 in, 1 out]
      }
      frame False {
        n36 = Format Into String(format string=w85, initial string=w81, w83, w84, w82, w84) -> (resulting string=w80:string)  [unwired: 1 in, 1 out]
      }
    }
  }
  n37 = Search and Replace String(input string=w9, search string="[''']" ("regular expression"), replace string="[\"'\"]" ("regular expression")) -> (result string=w6:string)  [unwired: 5 in, 3 out]
  n38 = Search and Replace String(input string=w6, search string="['\\']" ("regular expression"), replace string="['\\\\']" ("regular expression")) -> (result string=→"regular expression":string)  [unwired: 5 in, 3 out]
